vi "obtainQueue.vi"(8 "Error In":errorcluster) -> (0 "Error Out":errorcluster, 3 "MissionQueue.lvclass":refnum<class "MissionQueue.lvclass">)   [LabVIEW 2011, in "MissionQueue.lvclass"]
doc: "Obtain a reference to a newly created MissionQueue.\n\nAuthor: Jared Kirschner"
uses:
  MissionQueue.lvclass
  Missions/GenericMission/GenericMission.lvclass
  MissionQueue.lvclass/MissionQueue.ctl
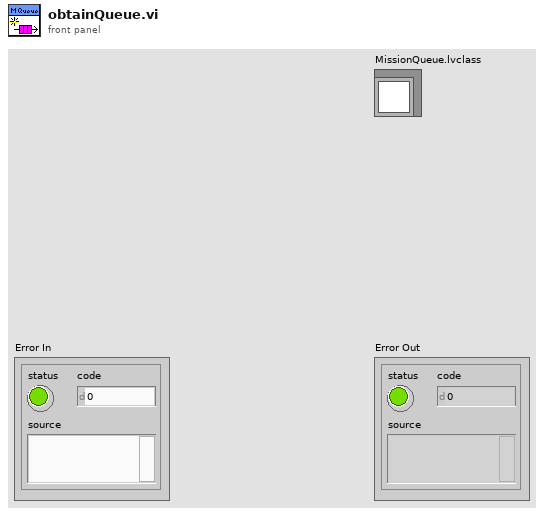
[diagram p1: front panel]
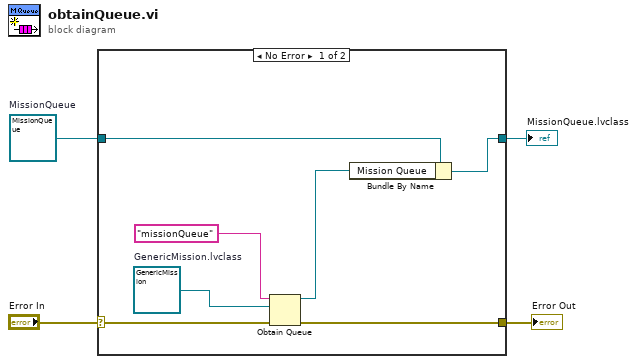
[diagram p0: block diagram]
diagram:
  w4 = refnum<class "MissionQueue.lvclass"> refnum  # MissionQueue
  n1 = case shown="No Error" "Error In" {
    selector: "Error In" -> [w11 w12]
    tunnel: w4 -> [w9 w13]
    tunnel: [w8 w13] -> w2
    tunnel: [w6 w12] -> w1
    frame No Error {
      w7 = refnum<class "GenericMission.lvclass"> refnum  # GenericMission.lvclass
      n2 = Obtain Queue(name (unnamed)="missionQueue", element data type=w7, error in (no error)=w11) -> (queue out=w5:refnum<queue>, error out=w6:errorcluster)  [unwired: 2 in, 1 out]
      n3 = Bundle By Name(cluster=w9, "Mission Queue"=w5) -> (w8:refnum<class "MissionQueue.lvclass">)
    }
    frame Error {
    }
  }
  "Error Out" <- w1
  "MissionQueue.lvclass" <- w2
